vi "Configure Dialog.vi"(8 "Error In":errorcluster, 11 "Undeploy Libraries Msg in":refnum<class "Undeploy Libraries Msg.lvclass">) -> (0 "Error Out":errorcluster, 2 "OK?":bool, 3 "Undeploy Libraries Msg out":refnum<class "Undeploy Libraries Msg.lvclass">)   [LabVIEW 2015, in "CS++DSCManager.lvlib" / "Undeploy Libraries Msg.lvclass"]
doc: "This overrides of this dynamic dispatch VI open the frontpanel to set derived message attributes."
uses:
  Undeploy Libraries Msg.lvclass
  Undeploy Libraries Msg.lvclass/Undeploy Libraries Msg.ctl
panel:
  in  "OK":bool
  in  "Cancel":bool
  in  "Library Paths":path[](array[path])
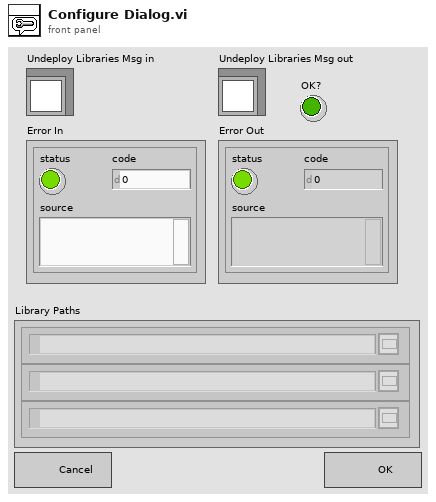
[diagram p1: front panel]
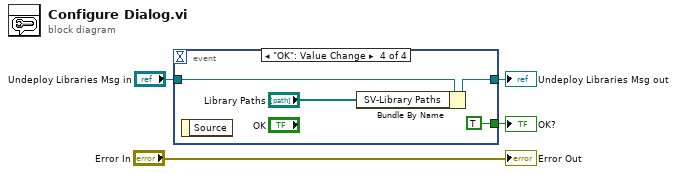
[diagram p0: block diagram]
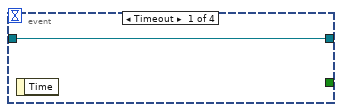
[diagram p2: hidden frame]
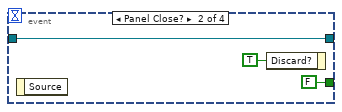
[diagram p3: hidden frame]
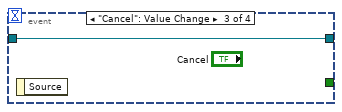
[diagram p4: hidden frame]
diagram:
  n1 = event shown="[3] \"OK\": Value Change" {
    selector: _ -> [_ _ _ _]
    dyn-events: _ -> [_ _ _ _]
    timeout: _ -> [_ _ _ _]
    tunnel: [w5 w6 w9 w12] -> w2
    tunnel: "Undeploy Libraries Msg in" -> [w5 w6 w9 w13]
    tunnel: [_ FALSE _ TRUE] -> w1
    event Timeout {
      n2 = event-data() -> ()  [unwired: 1 in, 1 out]
    }
    event Panel Close? {
      n3 = event-data() -> ()  [unwired: 1 in, 1 out]
      n4 = event-data("Discard?"=TRUE) -> ()  [unwired: 1 in, 1 out]
    }
    event "Cancel": Value Change {
      n5 = event-data() -> ()  [unwired: 1 in, 1 out]
    }
    event "OK": Value Change {
      n6 = event-data() -> ()  [unwired: 1 in, 1 out]
      n7 = Bundle By Name(cluster=w13, "SV-Library Paths"="Library Paths") -> (w12:refnum<class "Undeploy Libraries Msg.lvclass">)
    }
  }
  "Undeploy Libraries Msg out" <- w2
  "OK?" <- w1
  "Error Out" <- "Error In"
